vi "Check Status.vi"(8 "error in (no error)":errorcluster, 9 "channel (1)":u8=1 min=1 max=4 step=1, 10 "status register (T:present)":bool=TRUE, 11 "VISA resource name":refnum<visa-resource-name>) -> (0 "error out":errorcluster, 1 "value":i32, 3 "VISA resource name out":refnum<visa-resource-name>)   [LabVIEW 2020, in "Agilent 6XXX Series.lvlib"]
doc: "This function reads the status register which indicates the present state of the instrument or the accumulated status register which indicates all the conditions that have occurred since it was last read."
uses:
  <instrlib>/Agilent 6XXX Series/Agilent 6XXX Series.lvlib
panel:
  # "present state"
  # "accumulated"
  # "*662xA only"
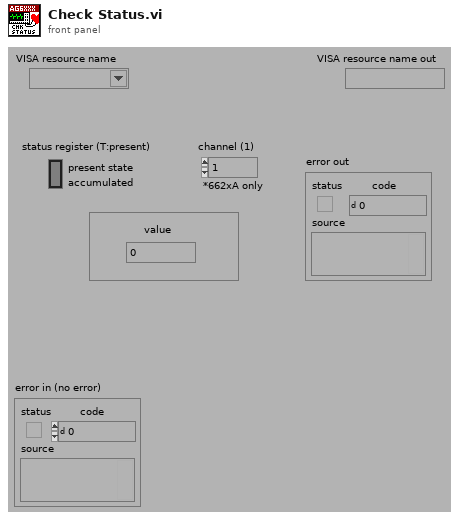
[diagram p1: front panel]
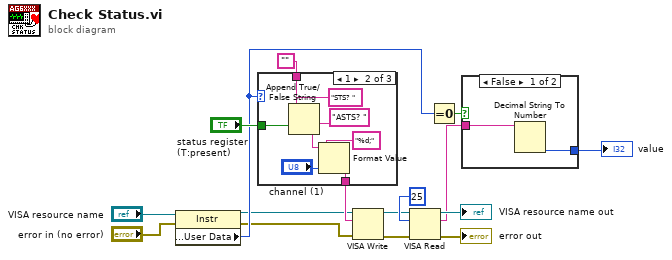
[diagram p0: block diagram]
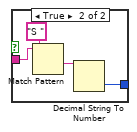
[diagram p2: hidden frame]
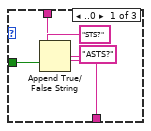
[diagram p3: hidden frame]
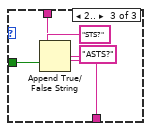
[diagram p4: hidden frame]
diagram:
  n1 = property class="Instr"(reference="VISA resource name", error in="error in (no error)") -> (reference out=w4:refnum<visa-resource-name>, error out=w3:errorcluster, "General Settings:User Data"=w7:u32)
  n2 = case shown="1" w7 {
    tunnel: "" -> [w19 w27 w32]
    tunnel: [w17 w24 w30] -> w11
    tunnel: "status register (T:present)" -> [w18 w22 w31]
    frame ..0 {
      n3 = Append True/False String(1:w18, 2:"ASTS?", 3:"STS?", 4:w19) -> (0:w17:string)
    }
    frame 1 {
      n4 = Append True/False String(1:w22, 2:"ASTS? ", 3:"STS? ", 4:w27) -> (0:w26:string)
      n5 = Format Value(string ("")=w26, format string="%d;", value (0)="channel (1)") -> (output string=w24:string)
    }
    frame 2.. {
      n6 = Append True/False String(1:w31, 2:"ASTS?", 3:"STS?", 4:w32) -> (0:w30:string)
    }
  }
  n7 = VISA Write(VISA resource name=w4, write buffer=w11, error in (no error)=w3) -> (VISA resource name out=w1:refnum<visa-resource-name>, error out=w2:errorcluster)  [unwired: 1 out]
  n8 = VISA Read(VISA resource name=w1, byte count=u32 25, error in (no error)=w2) -> (VISA resource name out=→"VISA resource name out":refnum<visa-resource-name>, read buffer=w9:string, error out=→"error out":errorcluster)  [unwired: 1 out]
  n9 = Equal To 0?(x=w7) -> (x = 0?=w10:bool)
  n10 = case shown="False" w10 {
    tunnel: w9 -> [w36 w38]
    tunnel: [w35 w37] -> w8
    frame False {
      n11 = Decimal String To Number(string=w36) -> (number=w35:i32)  [unwired: 2 in, 1 out]
    }
    frame True {
      n12 = Match Pattern(string=w38, regular expression="S ") -> (after substring=w40:string)  [unwired: 1 in, 3 out]
      n13 = Decimal String To Number(string=w40) -> (number=w37:i32)  [unwired: 2 in, 1 out]
    }
  }
  "value" <- w8
